vi "Handle VI Settings.vi"(7 "Write VI? (F:Read)":bool, 8 "error in (no error)":errorcluster, 10 "VI Refnum":refnum<vi>, 11 "Save Restore Settings in":refnum<class "Save Restore Settings.lvclass">) -> (0 "error out":errorcluster, 3 "Save Restore Settings out":refnum<class "Save Restore Settings.lvclass">)   [LabVIEW 2016, in "Save Restore Settings.lvclass"]
doc: "Retrieves properties from the specified VI and stores them in the class.\n\nAuthored by Shawn Walpole\nsupport@mooregoodideas.com\nwww.mooregoodideas.com\n\nCopyright (c) 2010, Moore Good Ideas, Inc.\n\nAll rights reserved.\n\nRedistribution and use in source and binary forms, with or without modification, are permitted provided that the following conditions are met:\n\n * Redistributions of source code must retain the above copyright notice, this list of conditions and the following disclaimer.\n * Redistributions in binary form must reproduce the above copyright notice, this list of conditions and the following disclaimer in the documentation and/or other materials provided with the distribution.\n * Neither the name of Moore Good Ideas, Inc. nor the names of its contributors may be used to endorse or promote products derived from this software without specific prior written permission.\n\nTHIS SOFTWARE IS PROVIDED BY THE COPYRIGHT HOLDERS AND CONTRIBUTORS \"AS IS\" AND ANY EXPRESS OR IMPLIED WARRANTIES, INCLUDING, BUT NOT LIMITED TO, THE IMPLIED WARRANTIES OF MERCHANTABILITY AND FITNESS FOR A PARTICULAR PURPOSE ARE DISCLAIMED. IN NO EVENT SHALL THE COPYRIGHT OWNER OR CONTRIBUTORS BE LIABLE FOR ANY DIRECT, INDIRECT, INCIDENTAL, SPECIAL, EXEMPLARY, OR CONSEQUENTIAL DAMAGES (INCLUDING, BUT NOT LIMITED TO, PROCUREMENT OF SUBSTITUTE GOODS OR SERVICES; LOSS OF USE, DATA, OR PROFITS; OR BUSINESS INTERRUPTION) HOWEVER CAUSED AND ON ANY THEORY OF LIABILITY, WHETHER IN CONTRACT, STRICT LIABILITY, OR TORT (INCLUDING NEGLIGENCE OR OTHERWISE) ARISING IN ANY WAY OUT OF THE USE OF THIS SOFTWARE, EVEN IF ADVISED OF THE POSSIBILITY OF SUCH DAMAGE."
uses:
  <userlib>/_MGI/Application Control/MGI Save Restore Settings/Save Restore Settings.lvclass
  <vilib>/Utility/miscctls.llb/LVRectTypeDef.ctl
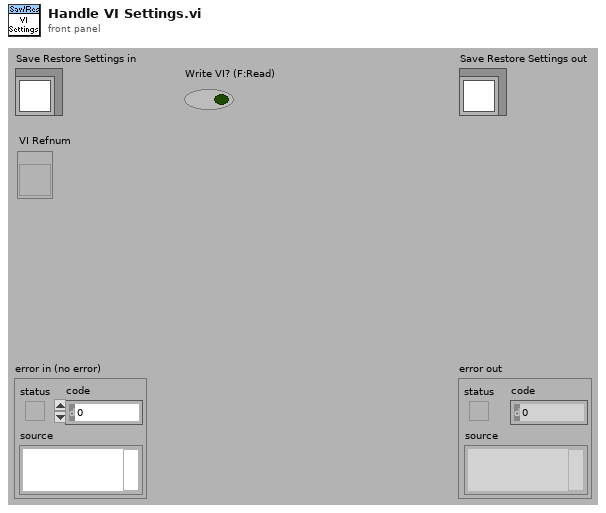
[diagram p1: front panel]
types:
  T1 = typedef "LVRectTypeDef.ctl" = cluster{"Left":i16, "Top":i16, "Right":i16, "Bottom":i16}
  T2 = cluster{"Left":i16, "Top":i16, "Right":i16, "Bottom":i16}
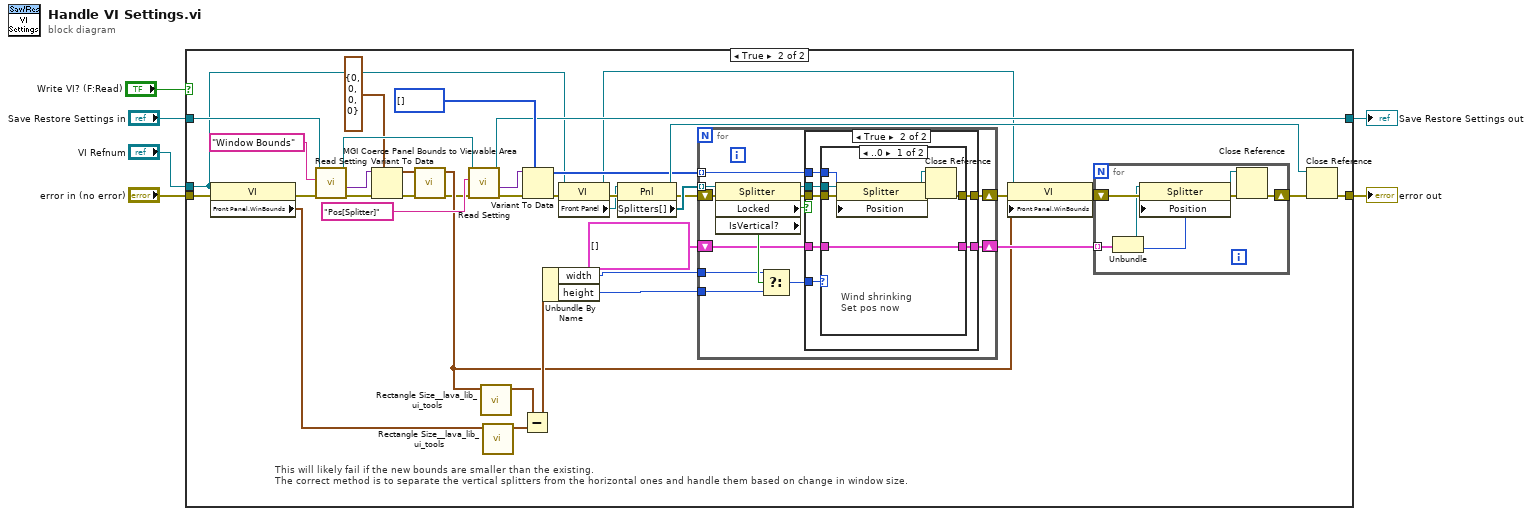
[diagram p0: block diagram]
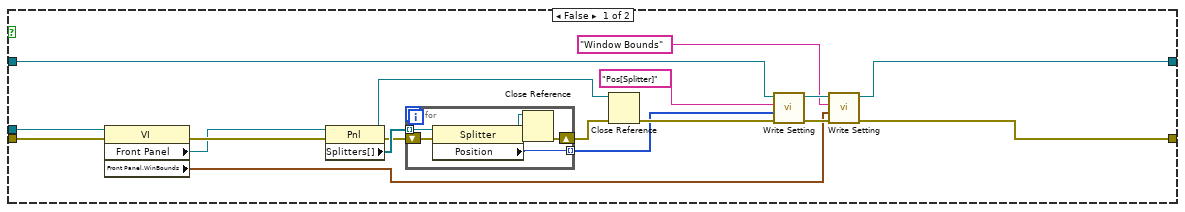
[diagram p2: hidden frame]
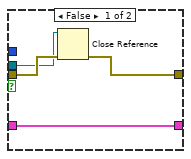
[diagram p3: hidden frame]
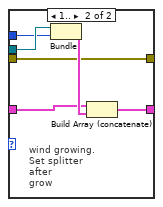
[diagram p4: hidden frame]
diagram:
  n1 = case shown="True" "Write VI? (F:Read)" {
    tunnel: "VI Refnum" -> [w22 w49]
    tunnel: "error in (no error)" -> [w21 w48]
    tunnel: "Save Restore Settings in" -> [w15 w51]
    tunnel: [w12 w52] -> w4
    tunnel: [w11 w50] -> w3
    frame False {
      n2 = property class="VI"(reference=w22, error in=w21) -> (error out=w18:errorcluster, "Front Panel"=w17:refnum<vi>, "Front Panel.WinBounds"=w7:T1)  [unwired: 1 out]
      n3 = property class="Pnl"(reference=w17, error in=w18) -> (reference out=w19:refnum<vi>, error out=w23:errorcluster, "Splitters[]"=w24:refnum<vi>[])
      n4 = for {
        tunnel: w24 -> [w29] mode=indexing
        tunnel: [w28] -> w9 mode=indexing
        shift-right: [w25] -> w20
        shift-left: w23 -> [w30]
        n5 = property class="Splitter"(reference=w29, error in=w30) -> (reference out=w27:refnum<vi>, error out=w26:errorcluster, "Position"=w28:i32)
        n6 = Close Reference(reference=w27, error in (no error)=w26) -> (error out=w25:errorcluster)
      }
      n7 = Close Reference(reference=w19, error in (no error)=w20) -> (error out=w16:errorcluster)
      n8 = call-dynamic "Write Setting.vi"("error in (no error)"=w16, "Tag Attribute"=w9, "Tag Name"="Pos[Splitter]", "Save Restore Settings in"=w15) -> ("error out"=w14:errorcluster, "Save Restore Settings out"=w13:refnum<class "Save Restore Settings.lvclass">)  [unwired: 6 in]
      n9 = call-dynamic "Write Setting.vi"("error in (no error)"=w14, "Tag Attribute"=w7, "Tag Name"="Window Bounds", "Save Restore Settings in"=w13) -> ("error out"=w12:errorcluster, "Save Restore Settings out"=w11:refnum<class "Save Restore Settings.lvclass">)  [unwired: 6 in]
    }
    frame True {
      # "This will likely fail if the new bounds are smaller than the existing.\nThe correct method is to separate the vertical splitters from the horizontal ones and handle them based on change in window size."
      n10 = property class="VI"(reference=w49, error in=w48) -> (error out=w47:errorcluster, "Front Panel.WinBounds"=w46:T1)  [unwired: 1 out]
      n11 = call-dynamic "Read Setting.vi"("error in (no error)"=w47, "Tag Name"="Window Bounds", "Save Restore Settings in"=w51) -> ("error out"=w60:errorcluster, "Tag Attribute"=w59:variant, "Save Restore Settings out"=w62:refnum<class "Save Restore Settings.lvclass">)  [unwired: 6 in]
      n12 = Variant To Data(error in=w60, type=T1 {"Left"=0, "Top"=0, "Right"=0, "Bottom"=0} ("Front Panel Window:Window Bounds"), Variant=w59) -> (data=w34:T1, error out=w31:errorcluster)
      n13 = call <userlib>:"MGI Coerce Panel Bounds to Viewable Area.vi"("Error In"=w31, "Panel Bounds In"=w34) -> ("Error Out"=w32:errorcluster, "Panel Bounds Out"=w33:T2)  [unwired: 8 in]
      n14 = call-dynamic "Read Setting.vi"("error in (no error)"=w32, "Tag Name"="Pos[Splitter]", "Save Restore Settings in"=w62) -> ("error out"=w57:errorcluster, "Tag Attribute"=w56:variant, "Save Restore Settings out"=w50:refnum<class "Save Restore Settings.lvclass">)  [unwired: 6 in]
      n15 = call <vilib>:"Rectangle Size__lava_lib_ui_tools.vi"("Rectangle"=w33) -> ("Rect Size"=w45:cluster{"width":i32, "height":i32})  [unwired: 8 in, 2 out]
      n16 = call <vilib>:"Rectangle Size__lava_lib_ui_tools.vi"("Rectangle"=w46) -> ("Rect Size"=w44:cluster{"width":i32, "height":i32})  [unwired: 8 in, 2 out]
      n17 = Subtract(x=w45, y=w44) -> (x-y=w39:cluster{"width":i32, "height":i32})
      n18 = Variant To Data(error in=w57, type=i32[] [], Variant=w56) -> (data=w53:i32[], error out=w54:errorcluster)
      n19 = Unbundle By Name(w39) -> ("width"=w38:i32, "height"=w37:i32)
      n20 = property class="VI"(reference=w49, error in=w54) -> (reference out=w42:refnum<vi>, error out=w65:errorcluster, "Front Panel"=w64:refnum<vi>)
      n21 = property class="Pnl"(reference=w64, error in=w65) -> (reference out=w66:refnum<vi>, error out=w67:errorcluster, "Splitters[]"=w68:refnum<vi>[])
      n22 = for {
        tunnel: w68 -> [w87] mode=indexing
        tunnel: w53 -> [w77] mode=indexing
        shift-right: [w80] -> w43
        shift-left: w67 -> [w88]
        tunnel: w38 -> [w85]
        tunnel: w37 -> [w84]
        shift-right: [w78] -> w35
        shift-left: cluster{refnum<vi>, "Position":i32}[] [] -> [w79]
        n23 = property class="Splitter"(reference=w87, error in=w88) -> (reference out=w81:refnum<vi>, error out=w82:errorcluster, "Locked"=w83:bool, "IsVertical?"=w86:bool)
        n24 = Select(t=w85, s=w86, f=w84) -> (s? t:f=w76:i32)
        n25 = case shown="True" w83 {
          tunnel: w82 -> [w92 w94]
          tunnel: w81 -> [w91 w98]
          tunnel: [w90 w93] -> w80
          tunnel: w79 -> [w89 w95]
          tunnel: [w89 w96] -> w78
          tunnel: w76 -> [_ w99]
          tunnel: w77 -> [_ w97]
          frame False {
            n26 = Close Reference(reference=w91, error in (no error)=w92) -> (error out=w90:errorcluster)
          }
          frame True {
            n27 = case shown="..0" w99 {
              tunnel: w98 -> [w104 w112]
              tunnel: w97 -> [w103 w111]
              tunnel: [w106 w109] -> w96
              tunnel: w95 -> [w106 w108]
              tunnel: w94 -> [w105 w107]
              tunnel: [w101 w107] -> w93
              frame ..0 {
                # "Wind shrinking\nSet pos now"
                n28 = property class="Splitter"(reference=w104, error in=w105, "Position"=w103) -> (reference out=w102:refnum<vi>, error out=w100:errorcluster)
                n29 = Close Reference(reference=w102, error in (no error)=w100) -> (error out=w101:errorcluster)
              }
              frame 1.. {
                # "wind growing.\nSet splitter after\ngrow"
                n30 = Bundle(w112, "Position"=w111) -> (w110:cluster{refnum<vi>, "Position":i32})  [unwired: 1 in]
                n31 = Build Array (concatenate)(w108, w110) -> (w109:cluster{refnum<vi>, "Position":i32}[])
              }
            }
          }
        }
      }
      n32 = property class="VI"(reference=w42, error in=w43, "Front Panel.WinBounds"=w33) -> (error out=w41:errorcluster)  [unwired: 1 out]
      n33 = for {
        shift-right: [w72] -> w40
        shift-left: w41 -> [w75]
        tunnel: w35 -> [w71] mode=indexing
        n34 = Unbundle(w71) -> (w70:refnum<vi>, "Position"=w69:i32)
        n35 = property class="Splitter"(reference=w70, error in=w75, "Position"=w69) -> (reference out=w73:refnum<vi>, error out=w74:errorcluster)
        n36 = Close Reference(reference=w73, error in (no error)=w74) -> (error out=w72:errorcluster)
      }
      n37 = Close Reference(reference=w66, error in (no error)=w40) -> (error out=w52:errorcluster)
    }
  }
  "error out" <- w4
  "Save Restore Settings out" <- w3
